vi "3 Mirrors Make Waveforms.vi"(0 "Axis Voltage Data":T1, 5 "Mirror Coupling":dbl, 7 "Phase 01":dbl, 9 "Phase 02":dbl, 11 "Phase 03":dbl) -> (8 "Waveform Data":waveform(dbl)[](array[waveform]), 15 "Error Out":errorcluster)   [LabVIEW 2020]
uses:
  3 Mirror Scan Type Defs/3 Mirror Scan ROI Voltage Data.ctl
  <vilib>/measure/NI_MABase.lvlib
panel:
  out "Y Axis 02":waveform(dbl)(graph)
  out "Y Axis 01":waveform(dbl)(graph)
  out "X Axis":waveform(dbl)(graph)
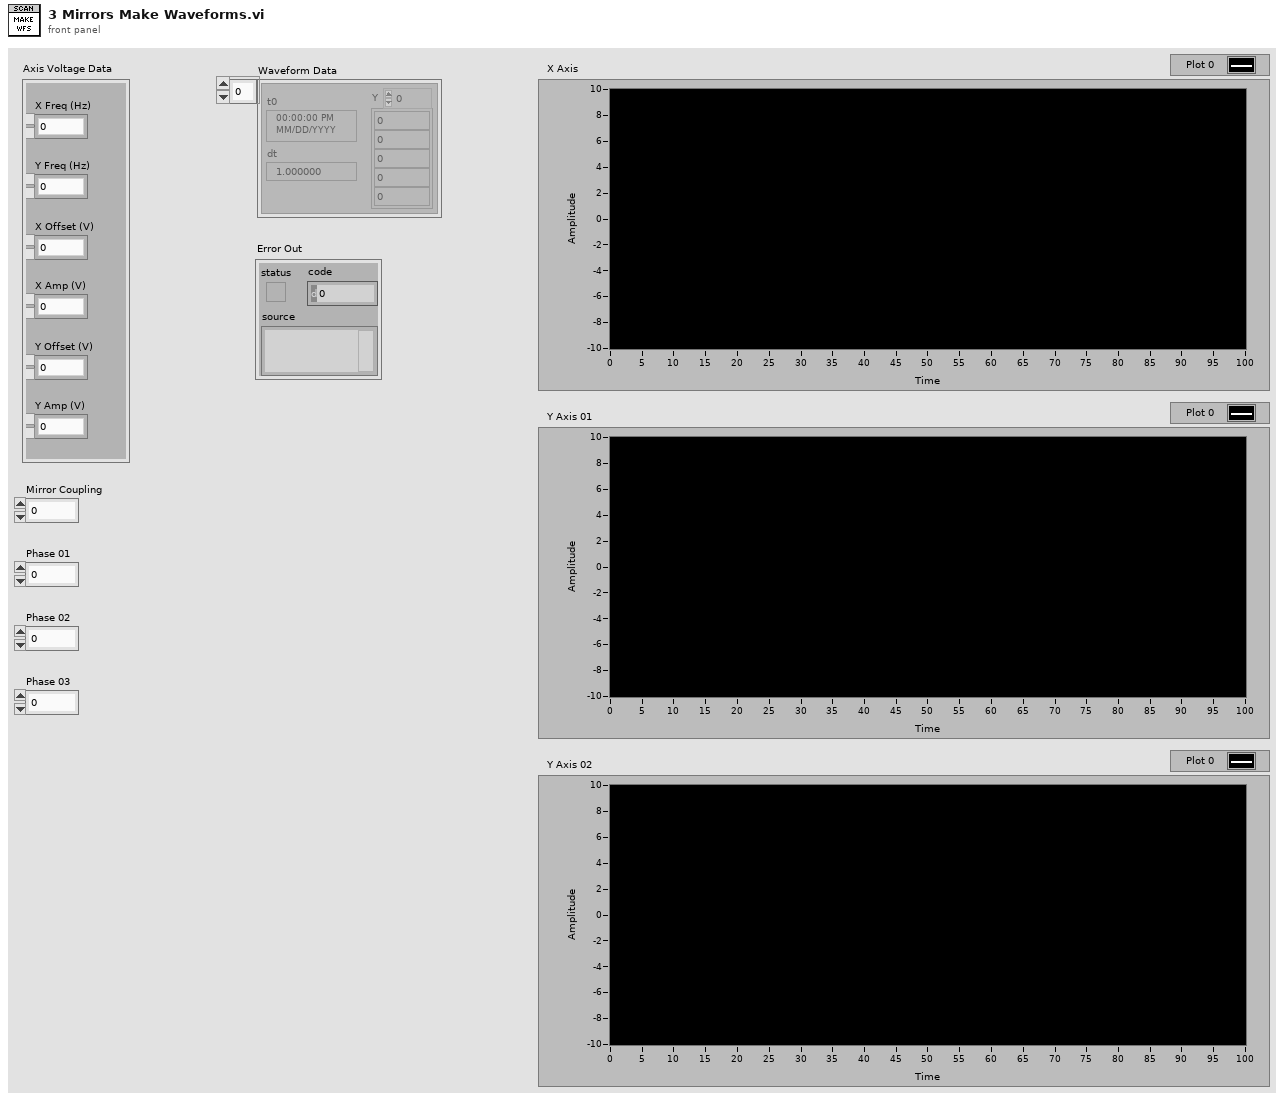
[diagram p1: front panel]
types:
  T1 = typedef "3 Mirror Scan ROI Voltage Data.ctl" = cluster{"X Freq (Hz)":dbl, "Y Freq (Hz)":dbl, "X Offset (V)":dbl, "X Amp (V)":dbl, "Y Offset (V)":dbl, "Y Amp (V)":dbl}
  T2 = enum16{"Sine Wave", "Triangle Wave", "Square Wave", "Sawtooth Wave"}
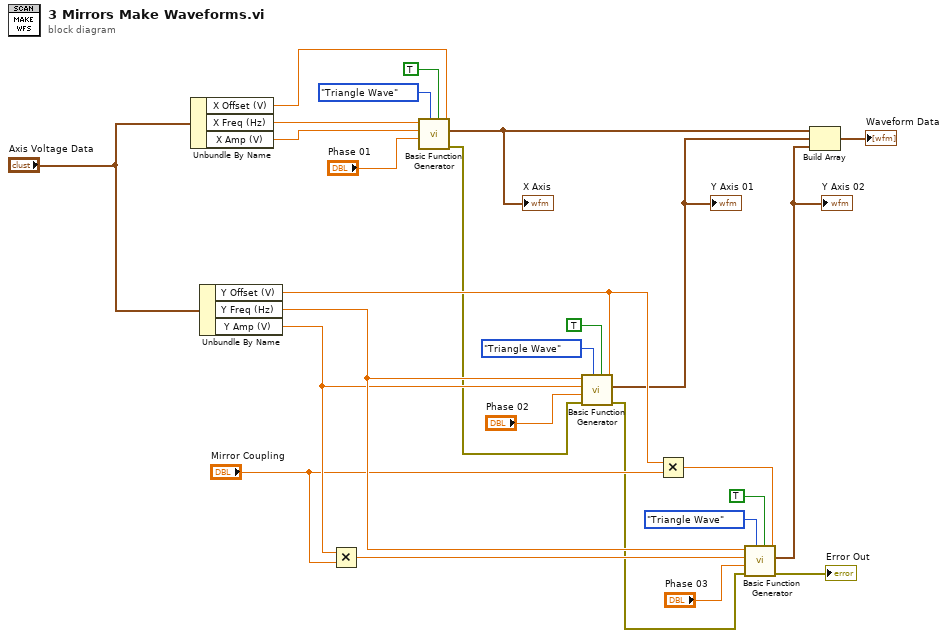
[diagram p0: block diagram]
diagram:
  n1 = Unbundle By Name("Axis Voltage Data") -> ("X Offset (V)"=w22:dbl, "X Freq (Hz)"=w24:dbl, "X Amp (V)"=w23:dbl)
  n2 = Unbundle By Name("Axis Voltage Data") -> ("Y Offset (V)"=w14:dbl, "Y Freq (Hz)"=w15:dbl, "Y Amp (V)"=w12:dbl)
  n3 = Multiply(x=w12, y="Mirror Coupling") -> (x*y=w11:dbl)
  n4 = call <vilib>:"Basic Function Generator.vi"("offset"=w22, "reset signal"=TRUE, "signal type"=T2."Triangle Wave", "phase"="Phase 01", "amplitude"=w23, "frequency"=w24) -> ("error out"=w7:errorcluster, "signal out"=w3:waveform(dbl))  [unwired: 3 in, 1 out]
  "X Axis" <- w3
  n5 = call <vilib>:"Basic Function Generator.vi"("offset"=w14, "reset signal"=TRUE, "signal type"=T2."Triangle Wave", "error in (no error)"=w7, "phase"="Phase 02", "amplitude"=w12, "frequency"=w15) -> ("error out"=w8:errorcluster, "signal out"=w2:waveform(dbl))  [unwired: 2 in, 1 out]
  "Y Axis 01" <- w2
  n6 = Multiply(x=w14, y="Mirror Coupling") -> (x*y=w13:dbl)
  n7 = call <vilib>:"Basic Function Generator.vi"("offset"=w13, "reset signal"=TRUE, "signal type"=T2."Triangle Wave", "error in (no error)"=w8, "phase"="Phase 03", "amplitude"=w11, "frequency"=w15) -> ("error out"=→"Error Out":errorcluster, "signal out"=w1:waveform(dbl))  [unwired: 2 in, 1 out]
  "Y Axis 02" <- w1
  n8 = Build Array(w3, w2, w1) -> (→"Waveform Data":waveform(dbl)[])
